vi "SAOMM-HistoParser.vi"(7 "DataStream":u8[](array[numeric])=[60, 0, 0, 0, 0, 0, 0, 0, 29, 105, 134, 205, 0, 0, 0, 0, 0, 0, 0, 0, 0, 0, 240, 63, 0, 0, 0, 0, 0, 0, 0, 64, 0, 0, 0, 0, 0, 0, 8, 64, 1, 0, 0, 0, 5, 0, 0, 0, 6, 0, 0, 0, 7, 0, 0, 0, 8, 0, 0, 0, 0, 0, 0, 0, 0, 0, 34, 64, 0, 0, 0, 0, 0, 0, 36, 64, 0, 0, 0, 0, 0, 0, 38, 64, 0, 0, 0, 0, 0, 0, 40, 64, 0, 0, 0, 0, 0, 0, 42, 64, 0, 0, 0, 0, 0, 0, 44, 64, 0, 0, 0, 0, 0, 0, 46, 64, 0, 0, 0, 0, 0, 0, 0, 0, 0, 0, 0, 0, 0, 0, 0, 0, 0, 0, 0, 0, 0, 0, 0, 0, 0, 0, 0, 0, 0, 0, 0, 0, 0, 0, 0, 0, 0, 0, 0, 0, 0, 0, 0, 0, 0, 0, 0, 0, 0, 0, 0, 0, 0, 0, 0, 0, 0, 0, 0, 0, 0, 0, 0, 0, 0, 0, 0, 0, 0, 0, 0, 0, 0, 0, 0, 0, 0, 0, 0, 0, 0, 0, 0, 0, 0, 0, 0, 0, 0, 0, 0, 0, 0, 0, 0, 0, 0, 0, 0, 0, 0, 0, 0, 0, 0, 0, 0, 0, 0, 0, 0, 0, 0, 0, 0, 0, 0, 0, 0, 0, 0, 0, 0, 0, 0, 0, 0, 0, 0, 0, 0, 0, 0, 0, 0, 0, 0, 0, 0, 0, 0, 0, 48, 64, 0, 0, 0, 0, 0, 0, 0, 0, 0, 0, 0, 0, 0, 0, 0, 0, 0, 0, 0, 0, 0, 0, 0, 0, 0, 0, 0, 0, 0, 0, 0, 0, 0, 0, 0, 0, 0, 0, 0, 0, 0, 0, 0, 0, 0, 0, 0, 0, 0, 0, 0, 0, 0, 0, 0, 0, 0, 0, 0, 0, 0, 0, 0, 0, 0, 0, 0, 0, 0, 0, 0, 0, 0, 0, 0, 0, 0, 0, 0, 0, 0, 0, 0, 0, 0, 0, 0, 0, 0, 0, 0, 0, 0, 0, 0, 0, 0, 0, 0, 0, 0, 0, 0, 0, 0, 0, 0, 0, 0, 0, 0, 0]) -> (6 "Source cluster":T2 {"SNR" format="%.32f"}, 10 "Hexapod cluster":T1 {"Hexapode_ServoY" format="%.6f"; "Hexapod_Console" format="%.6f"; "Hexapod_Position" format="%.6f"})   [LabVIEW 2011]
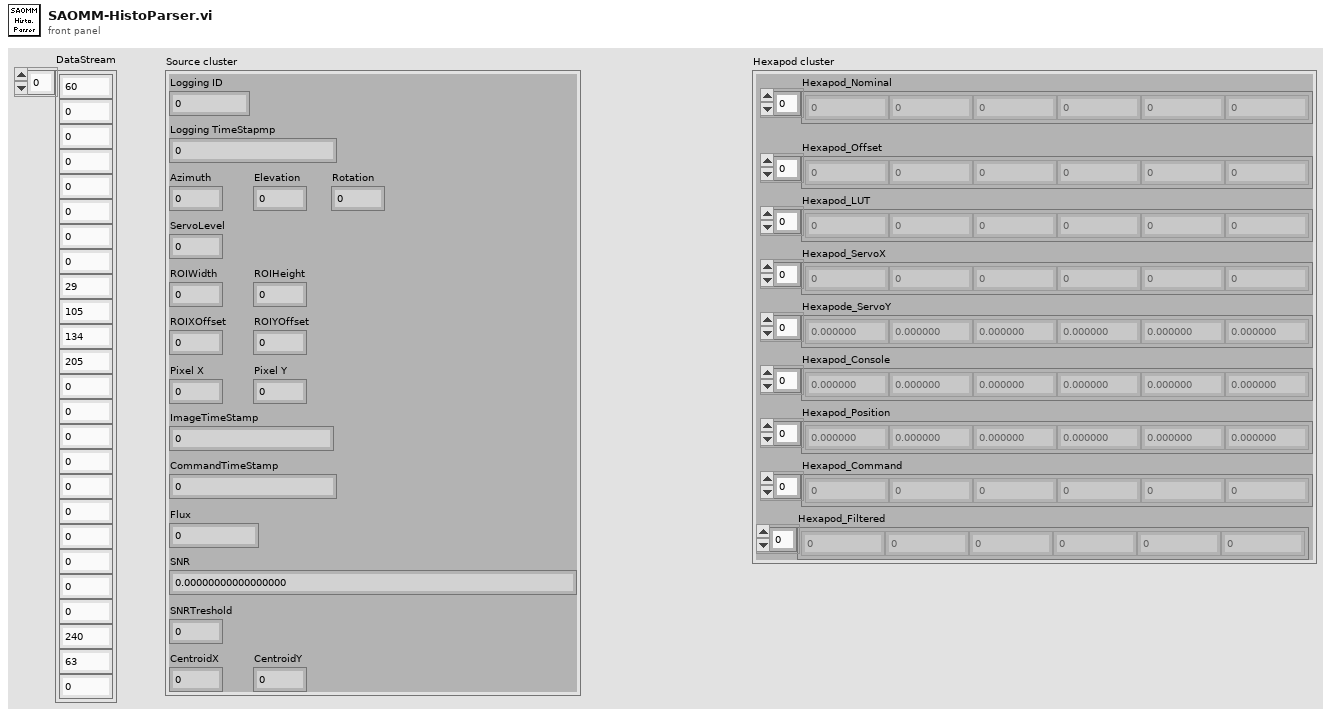
[diagram p1: front panel]
types:
  T1 = cluster{"Hexapod_Nominal":dbl[], "Hexapod_Offset":dbl[], "Hexapod_LUT":dbl[], "Hexapod_ServoX":dbl[], "Hexapode_ServoY":dbl[], "Hexapod_Console":dbl[], "Hexapod_Position":dbl[], "Hexapod_Command":dbl[], "Hexapod_Filtered":dbl[]}
  T2 = cluster{"Logging ID":u32, "Logging TimeStapmp":u64, "Azimuth":dbl, "Elevation":dbl, "Rotation":dbl, "ServoLevel":u16, "ROIWidth":u16, "ROIHeight":u16, "ROIXOffset":u16, "ROIYOffset":u16, "Pixel X":dbl, "Pixel Y":dbl, "ImageTimeStamp":u64, "CommandTimeStamp":u64, "Flux":dbl, "SNR":dbl, "SNRTreshold":dbl, "CentroidX":dbl, "CentroidY":dbl}
  T3 = cluster{u32, u64, dbl, dbl, dbl, u16, u16, u16, u16, u16, dbl, dbl, u64, u64, dbl, dbl, dbl, dbl, dbl}
  T4 = cluster{dbl[], dbl[], dbl[], dbl[], dbl[], dbl[], dbl[], dbl[], dbl[]}
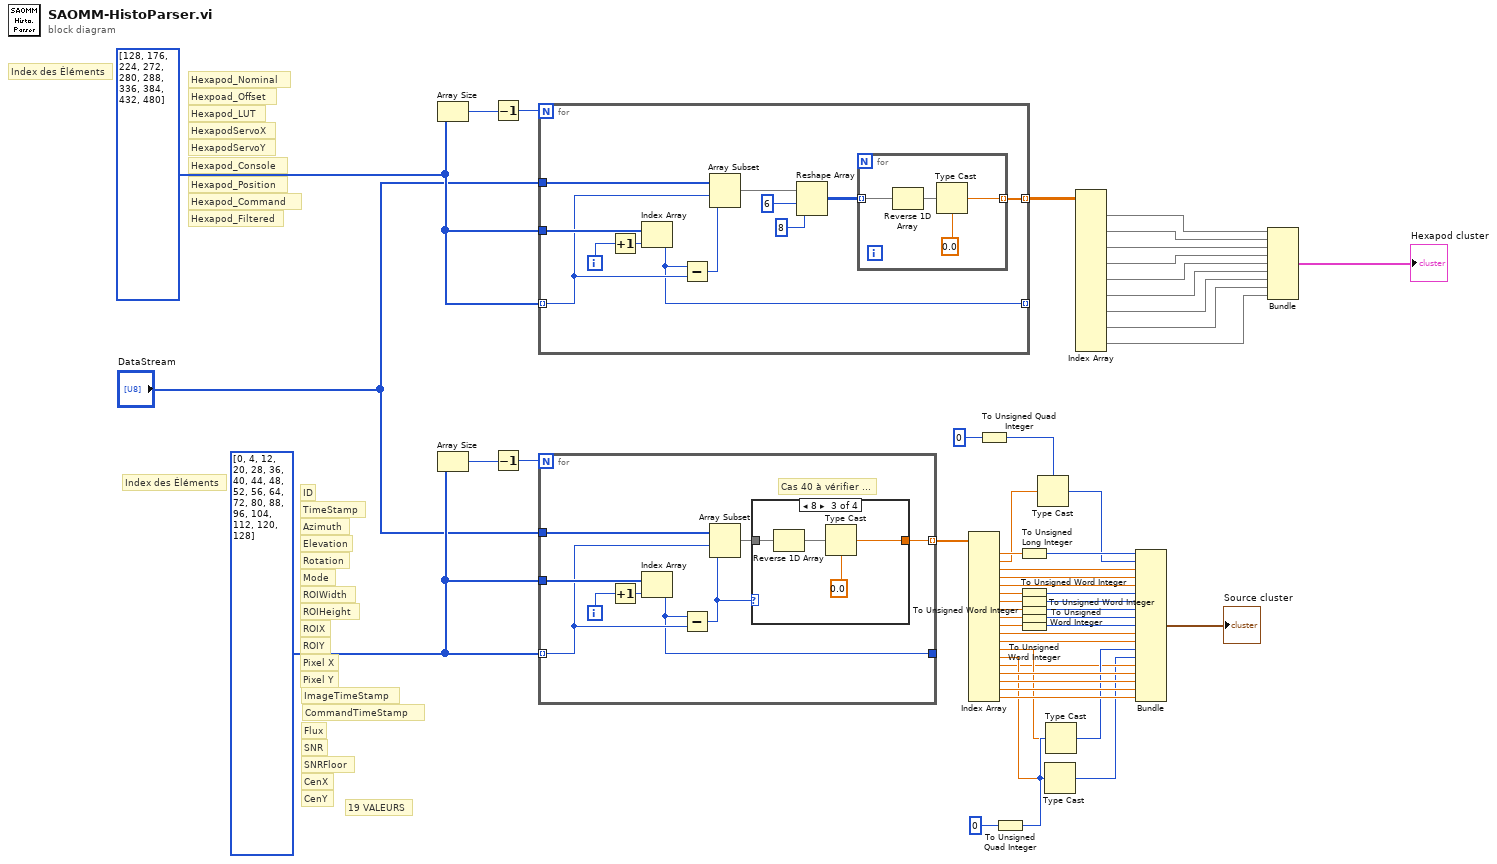
[diagram p0: block diagram]
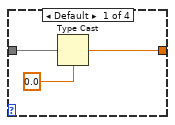
[diagram p2: hidden frame]
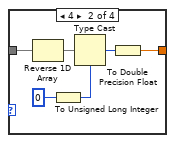
[diagram p3: hidden frame]
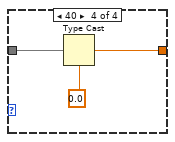
[diagram p4: hidden frame]
diagram:
  w51 = i32[] [128, 176, 224, 272, 280, 288, 336, 384, 432, 480]
  w52 = i32[] [0, 4, 12, 20, 28, 36, 40, 44, 48, 52, 56, 64, 72, 80, 88, 96, 104, 112, 120, 128]
  # "Hexapod_Filtered"
  # "Hexapod_Command"
  # "Hexapod_Position"
  # "Hexapod_Console"
  # "HexapodServoY"
  # "HexapodServoX"
  # "Hexapod_LUT"
  # "Hexpoad_Offset"
  # "Hexapod_Nominal"
  # "19 VALEURS"
  # "CommandTimeStamp"
  # "ImageTimeStamp"
  # "Index des Éléments"
  # "CenY"
  # "CenX"
  # "SNRFloor"
  # "SNR"
  # "Flux"
  # "Pixel Y"
  # "Pixel X"
  # "ROIY"
  # "ROIX"
  # "ROIHeight"
  # "ROIWidth"
  # "Mode"
  # "Rotation"
  # "Elevation"
  # "Azimuth"
  # "TimeStamp"
  # "ID"
  # "Index des Éléments"
  n1 = Array Size(array=w51) -> (size(s)=w36:i32)
  n2 = Array Size(array=w52) -> (size(s)=w39:i32)
  n3 = Decrement(x=w36) -> (x-1=w35:i32)
  n4 = Decrement(x=w39) -> (x-1=w38:i32)
  n5 = for {
    N: w35 -> [_]
    tunnel: "DataStream" -> [w64]
    tunnel: w51 -> [w58] mode=indexing
    tunnel: w51 -> [w61]
    tunnel: [w54] -> w34 mode=indexing
    tunnel: [w53] -> _ mode=indexing
    i -> [w62]
    n6 = Increment(x=w62) -> (x+1=w63:i32)
    n7 = Index Array(array=w61, index=w63) -> (element=w53:i32)
    n8 = Subtract(x=w53, y=w58) -> (x-y=w59:i32)
    n9 = Array Subset(array=w64, index=w58, length=w59) -> (w60:u8[])
    n10 = Reshape Array(w60, 6 ("dimension size"), 8 ("dimension size")) -> (w57:u8[][])
    n11 = for {
      tunnel: w57 -> [w66] mode=indexing
      tunnel: [w65] -> w54 mode=indexing
      n12 = Reverse 1D Array(array=w66) -> (reversed array=w68:u8[])
      n13 = Type Cast(type=0.0, x=w68) -> (*(type *) &x=w65:dbl)
    }
  }
  n14 = for {
    N: w38 -> [_]
    tunnel: "DataStream" -> [w77]
    tunnel: w52 -> [w70] mode=indexing
    tunnel: w52 -> [w74]
    tunnel: [w71] -> w37 mode=indexing
    tunnel: [w69] -> _
    i -> [w75]
    # "Cas 40 à vérifier ..."
    n15 = Increment(x=w75) -> (x+1=w76:i32)
    n16 = Index Array(array=w74, index=w76) -> (element=w69:i32)
    n17 = Subtract(x=w69, y=w70) -> (x-y=w72:i32)
    n18 = Array Subset(array=w77, index=w70, length=w72) -> (w73:u8[])
    n19 = case shown="8" w72 {
      tunnel: w73 -> [w80 w82 w87 w92]
      tunnel: [w79 w83 w88 w91] -> w71
      frame Default {
        n20 = Type Cast(type=0.0, x=w80) -> (*(type *) &x=w79:dbl)
      }
      frame 4 {
        n21 = Reverse 1D Array(array=w82) -> (reversed array=w81:u8[])
        n22 = To Unsigned Long Integer(number=0) -> (unsigned 32bit integer=w85:u32)
        n23 = Type Cast(type=w85, x=w81) -> (*(type *) &x=w84:u32)
        n24 = To Double Precision Float(number=w84) -> (double precision float=w83:dbl)
      }
      frame 8 {
        n25 = Reverse 1D Array(array=w87) -> (reversed array=w90:u8[])
        n26 = Type Cast(type=0.0, x=w90) -> (*(type *) &x=w88:dbl)
      }
      frame 40 {
        n27 = Type Cast(type=0.0, x=w92) -> (*(type *) &x=w91:dbl)
      }
    }
  }
  n28 = Index Array(array=w37) -> (element #1=w23:dbl, element #2=w2:dbl, element #3=w24:dbl, element #4=w25:dbl, element #5=w26:dbl, element #6=w27:dbl, element #7=w28:dbl, element #8=w29:dbl, element #9=w30:dbl, element #10=w31:dbl, element #11=w32:dbl, element #12=w33:dbl, element #13=w14:dbl, element #14=w13:dbl, element #15=w11:dbl, element #16=w44:dbl, element #17=w43:dbl, element #18=w42:dbl, element #19=w41:dbl)  [unwired: 19 in]
  n29 = To Unsigned Quad Integer(1:u64 0 ("number")) -> (0:w4:u64)
  n30 = To Unsigned Quad Integer(1:u64 0 ("number")) -> (0:w15:u64)
  n31 = To Unsigned Long Integer(number=w23) -> (unsigned 32bit integer=w22:u32)
  n32 = To Unsigned Word Integer(number=w27) -> (unsigned 16bit integer=w21:u16)
  n33 = To Unsigned Word Integer(number=w28) -> (unsigned 16bit integer=w20:u16)
  n34 = To Unsigned Word Integer(number=w29) -> (unsigned 16bit integer=w19:u16)
  n35 = To Unsigned Word Integer(number=w30) -> (unsigned 16bit integer=w18:u16)
  n36 = To Unsigned Word Integer(number=w31) -> (unsigned 16bit integer=w17:u16)
  n37 = Type Cast(type=w4, x=w2) -> (*(type *) &x=w1:u64)
  n38 = Type Cast(type=w15, x=w13) -> (*(type *) &x=w10:u64)
  n39 = Type Cast(type=w15, x=w14) -> (*(type *) &x=w12:u64)
  n40 = Index Array(array=w34) -> (element #1=w50:dbl[], element #2=w49:dbl[], element #3=w48:dbl[], element #4=w47:dbl[], element #5=w46:dbl[], element #6=w45:dbl[], element #7=w8:dbl[], element #8=w7:dbl[], element #9=w6:dbl[])  [unwired: 18 in]
  n41 = Bundle(w22, w1, w24, w25, w26, w21, w20, w19, w18, w17, w32, w33, w12, w10, w11, w44, w43, w42, w41) -> (→"Source cluster":T3)  [unwired: 1 in]
  n42 = Bundle(w50, w49, w48, w47, w46, w45, w8, w7, w6) -> (→"Hexapod cluster":T4)  [unwired: 1 in]
